vi "Gen - Text Wrapper.vi"(8 "Error In":errorcluster, 10 "Ref Listbox":refnum<vi>, 11 "Data in":string[][](array[string])) -> (0 "Error Out":errorcluster, 3 "Data Out":string[][](array[string]))   [LabVIEW 2020]
uses:
  <vilib>/Utility/miscctls.llb/LVRowAndColumnTypeDef.ctl
panel:
  out "# Items wrapped":i32
  out "Width Control":string
  in  "Width":u32
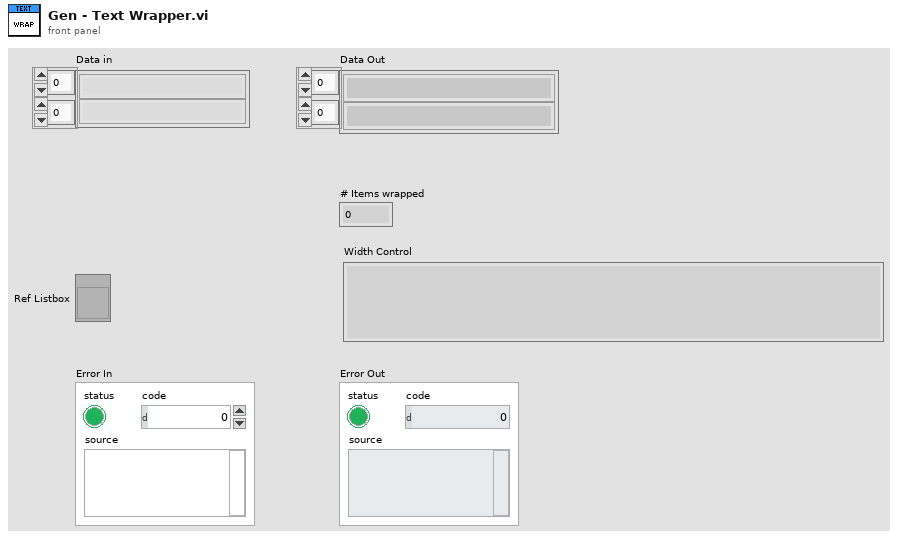
[diagram p1: front panel]
types:
  T1 = typedef "LVRowAndColumnTypeDef.ctl" = cluster{"Row":i32, "Column":i32}
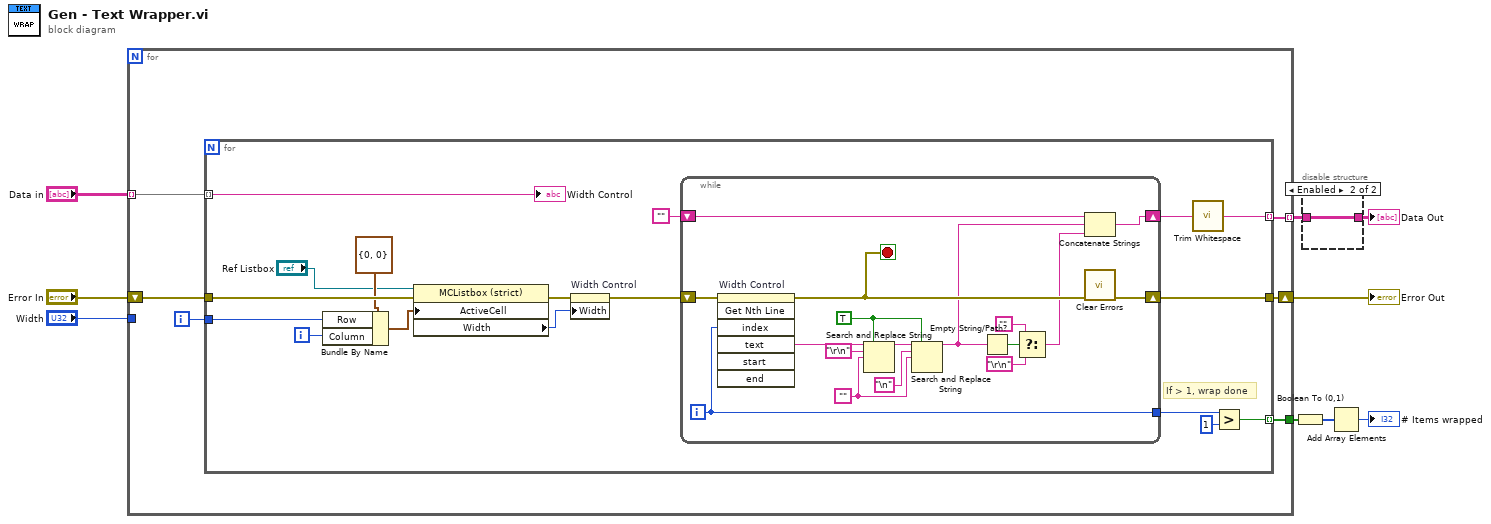
[diagram p0: block diagram]
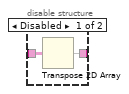
[diagram p2: hidden frame]
diagram:
  n1 = for {
    tunnel: "Width" -> [_]
    tunnel: [w13] -> w5
    tunnel: [w12] -> w2 mode=indexing
    tunnel: "Data in" -> [w11] mode=indexing
    shift-right: [w15] -> w9
    shift-left: "Error In" -> [w14]
    i -> [w10]
    n2 = for {
      tunnel: w14 -> [w23]
      tunnel: w11 -> [w30] mode=indexing
      tunnel: [w32] -> w15
      tunnel: [w27] -> w13 mode=indexing
      tunnel: [w24] -> w12 mode=indexing
      tunnel: w10 -> [w18]
      i -> [w19]
      # "If > 1, wrap done"
      n3 = Bundle By Name(cluster=T1 {"Row"=0, "Column"=0} ("Active Cell:Active Cell"), "Row"=w18, "Column"=w19) -> (w20:T1)
      n4 = property class="MCListbox (strict)"(reference="Ref Listbox", error in=w23, "ActiveCell"=w20) -> (error out=w22:errorcluster, "Width"=w16:u32)  [unwired: 1 out]
      n5 = property on="Width Control" class="Str"(error in=w22, "Width"=w16) -> (error out=w31:errorcluster)  [unwired: 1 in, 1 out]
      n6 = while {
        shift-right: [w47] -> w32
        shift-left: w31 -> [w49]
        tunnel: [w46] -> w28
        shift-right: [w42] -> w25
        shift-left: "" -> [w41]
        i -> [w46]
        stop <- w48 stop-if-true
        w37 = ""
        w39 = TRUE ("replace all? (F)")
        n7 = invoke on="Width Control" class="Str" method="Get Nth Line"(error in=w49, "index"=w46) -> (error out=w48:errorcluster, "text"=w33:string)  [unwired: 5 in, 5 out]
        n8 = Search and Replace String(replace all?=w39, input string=w33, search string="\r\n", replace string=w37) -> (result string=w38:string)  [unwired: 4 in, 3 out]
        n9 = Search and Replace String(replace all?=w39, input string=w38, search string="\n", replace string=w37) -> (result string=w34:string)  [unwired: 4 in, 3 out]
        n10 = Empty String/Path?(string/path=w34) -> (empty?=w45:bool)
        n11 = Select(t="", s=w45, f="\r\n") -> (s? t:f=w40:string)
        n12 = Concatenate Strings(w41, w34, w40) -> (w42:string)
        n13 = call <vilib>:"Clear Errors.vi"("error in (no error)"=w48) -> ("error out"=w47:errorcluster)  [unwired: 5 in, 1 out]
      }
      n14 = call <vilib>:"Trim Whitespace.vi"("string"=w25) -> ("trimmed string"=w24:string)  [unwired: 1 in]
      n15 = Greater?(x=w28, y=1) -> (0:w27:bool)
      "Width Control" <- w30
    }
  }
  "Error Out" <- w9
  n16 = Boolean To (0,1)(Boolean=w5) -> (0, 1=w6:i16[])
  n17 = disable-structure shown="Enabled" {
    disable-tunnel: w2 -> [w51 w52]
    disable-tunnel: [w50 w52] -> w1
    frame Disabled {
      n18 = Transpose 2D Array(2D array=w51) -> (transposed array=w50:string[][])
    }
    frame Enabled {
    }
  }
  "Data Out" <- w1
  n19 = Add Array Elements(numeric array=w6) -> (sum=→"# Items wrapped":i16)
